vi "AudioTest.Discrete Swept-Sine Measurements (Finite)_V2.vi"() -> ()   [LabVIEW 2018]
doc: "Overview:\nThis VI demonstrates simultaneous frequency response, level, and distortion measurements using a discrete swept-sine technique. This example implements analog input and analog output with 'Finite Samples' sample mode which minimizes sensitivity to bandwidth issues that can cause run-time errors when performing continuous measurements. This VI also demonstrates how finite acquisitions can be read in a single large block or in a series of smaller reads.\n\nRequirements:\nLabVIEW Full Development System\nSound and Vibration Toolkit\n\nInstructions:\n1. Connect the DUT to the DSA device.\n2. Select the AO excitation channel, AI stimulus channel, and AI response channel.\n3. Run the VI.\n\nDetails:\nThis VI performs a swept sine measurement to obtain the root-mean-square (RMS) levels of the acquired stimulus and response, the frequency response of the device under test (DUT), and the harmonic distortion on the response channel. You specify the source and measurement parameters, and the swept sine VIs handle all the DAQ-specific controls required to perform the measurement. You have direct control over the source, input, averaging, and display parameters. You also specify the engineering units to use for the swept sine measurements.\n\nYou can view the time records of the acquired stimulus and response signals. From these graphs, you can see that the transition to the next test frequency always occurs at a zero crossing to minimize non-linear disturbances to the DUT. The RMS levels, frequency response, and harmonic distortion are shown on different tabs."
uses:
  <vilib>/Utility/error.llb/DialogType.ctl
  <vilib>/addons/_NISVFA/_Generation/Signal Generation/SV Signal/SV Signal.lvclass/SV Signal.ctl
  <vilib>/addons/_NISVFA/_Generation/Signal Generation/SV Discrete Sweep/SV Discrete Sweep.lvclass/SV Discrete Sweep.ctl
  <vilib>/addons/Sound and Vibration/svt_Level/SVL AC & DC Level (Time) (1 Ch).vi
  <vilib>/addons/_NISVFA/_Shared subVIs/Common/SV Append Data (N Ch) (DBL).vi
  <vilib>/addons/_NISVFA/_Generation/Signal Generation/SV Signal/Write Leading Synchronization Pulse Enable.vi
  <vilib>/addons/_NISVFA/_Generation/Signal Generation/SV Discrete Sweep/Read All Frequencies and Amplitudes.vi
  <vilib>/addons/_NISVFA/_Generation/Signal Generation/SV Discrete Sweep/Write All Frequencies and Amplitudes.vi
  <vilib>/addons/_NISVFA/_Shared subVIs/Common/svc_Get SV Channel Info.vi
  <vilib>/Analysis/baseanly.llb/Mean.vi
  <vilib>/Analysis/baseanly.llb/Mean (DBL).vi
  <vilib>/addons/_NISVFA/_Shared subVIs/Windowing/svfa_Scaled Time Domain Window (Array).vi
  <vilib>/addons/_NISVFA/_Generation/Signal Generation/SV Discrete Sweep/Read Frequencies and Amplitudes.vi
  <vilib>/Analysis/4window.llb/Force Window.vi
  <vilib>/Analysis/4window.llb/Force Window (DBL).vi
  <vilib>/Analysis/4window.llb/Exponential Window.vi
  <vilib>/Analysis/4window.llb/Exponential Window (DBL).vi
  <vilib>/addons/_NISVFA/_Generation/Signal Generation/SV Discrete Sweep/SV Discrete Sweep.lvclass
  C:/Program Files (x86)/National Instruments/LabVIEW 2018/vi.lib/addons/_NISVFA/_Generation/Signal Generation/SV Signal/SV Signal.lvclass
  C:/Program Files (x86)/National Instruments/LabVIEW 2018/vi.lib/addons/_NISVFA/_Generation/Signal Generation/SV Function/SV Function.lvclass
  <vilib>/addons/_NISVFA/_Generation/Signal Generation/SV Discrete Sweep/Configure Frequency Sweep at Constant Amplitude.vi
  <vilib>/addons/_NISVFA/_Generation/Signal Generation/SV Signal/Write Ramp Parameters.vi
  <vilib>/addons/_NISVFA/_Generation/Signal Generation/SV Signal/Write DC Offset.vi
  <vilib>/addons/_NISVFA/_Generation/Signal Generation/SV Signal/Write Measurement Duration.vi
  <vilib>/addons/_NISVFA/_Generation/Signal Generation/SV Function/Write Measurement Cycles.vi
  <vilib>/addons/_NISVFA/_Generation/Signal Generation/SV Signal/Write Pre-Measurement Settling Duration.vi
  <vilib>/addons/_NISVFA/_Generation/Signal Generation/SV Function/Write Pre-Measurement Settling Cycles.vi
  <vilib>/addons/_NISVFA/_Generation/Signal Generation/SV Signal/Write Sample Rate.vi
  <vilib>/addons/_NISVFA/_Shared subVIs/Data Objects/Waveforms (DBL)/SV Read Next Measurement Data.vi
  <vilib>/addons/_NISVFA/_Shared subVIs/Common/svc_Get Window Info.vi
  <vilib>/addons/_NISVFA/_Shared subVIs/Common/svc_Unit Label to Engineering Units.vi
  <vilib>/addons/_NISVFA/_Shared subVIs/Common/svc_Engineering Units to Unit Label.vi
  <vilib>/addons/_NISVFA/_Spectrum Processing/subVIs/svfa_Spectrum Info Window to windowTd Type Def.vi
  <vilib>/Analysis/0measdsp.llb/Scaled Time Domain Window.vi
  <vilib>/Analysis/0measdsp.llb/Scaled Time Domain Window (DBL).vi
  <vilib>/Utility/error.llb/Error Cluster From Error Code.vi
  <vilib>/Analysis/baseanly.llb/Std Deviation and Variance.vi
  <vilib>/addons/_NISVFA/_Shared subVIs/Common/svc_Caller VI Returned in Error Source.vi
  <vilib>/addons/Sound and Vibration/svt_Single Tone Measurements/SVT Gain and Phase (Time).vi
  <vilib>/addons/Sound and Vibration/svt_Distortion/SVT THD and Harmonic Components (Frequency) (1 Ch).vi
  <vilib>/addons/_NISVFA/_Generation/Signal Generation/SV Signal/SV Signal.lvclass
  <vilib>/addons/_NISVFA/_Shared subVIs/Data Objects/Waveforms (DBL)/Waveforms (N Ch).lvclass
  <vilib>/addons/Sound and Vibration/svt_Distortion/SoundVib_Distortion.lvlib
  <vilib>/addons/Sound and Vibration/svt_Single Tone Measurements/SoundVib_SingleTone.lvlib
  Program Files (x86)/National Instruments/LabVIEW 2018/examples/Sound and Vibration/SoundVib_Audio Examples.lvlib
  C:/Program Files (x86)/National Instruments/LabVIEW 2018/vi.lib/addons/_NISVFA/_Generation/Signal Generation/SV Sinusoid/SV Sinusoid.lvclass
panel:
  in  "volume":dbl=40.0 format="%#_13g"
  in  "Play Cal Output":bool
  in  "Speaker Cal":path=path "C:/MTE/Utah Core Audio Test/Config/Speaker Calibration, PN XXX, SN YYY, v10-30-18.csv"
  out "Cal Speaker Out":waveform(dbl)(graph)
  out "Raw Mic":waveform(dbl)(graph)
  out "Mic dt":dbl
  out "Play dt":dbl
  out "Size Play":i32
  out "Size Mic":i32
  out "Data Cnt":i32
  out "Error":errorcluster
  out "Audio Error":errorcluster
  out "test time":u32
  in  "sweep settings":T1(tab)
  in  "device In":u32
  in  "device Out":u32=1
  in  "Samples/Sec":dbl=51200.0
  in  "Dur(s)":dbl=2.0 format="%.2p"
  out "CalcDur(s)":dbl=1.0 format="%.2p"
  in  "number of steps":i32=190 min=1
  in  "DC offset [V]":dbl format="%.2f"
  in  "amplitude [V]":dbl=1.0 format="%.2p"
  in  "frequency spacing":enum16{"Linear", "Logarithmic"}(ring)=enum."Logarithmic"
  in  "sweep range":cluster{"start":dbl, "stop":dbl}={"start"=20000.0, "stop"=100.0} {"stop" min=0.0 format="%.2f"; "start" min=0.0 format="%.2f"}
  in  "measurement":cluster{"time":dbl, "cycles":dbl}={"time"=0.001, "cycles"=10.0} {"cycles" min=5.0 max=1000.0 step=1.0; "time" min=0.0 max=5.0 step=0.0001 format="%.3f s"}
  in  "settling":cluster{"time":dbl, "cycles":dbl}={"time"=0.0, "cycles"=1.0} {"cycles" min=0.0 max=100.0 step=0.5; "time" min=0.0 max=5.0 step=0.0001 format="%.3f s"}
  in  "views":T2(tab)
  out "Response":waveform(dbl)[](graph)
  out "Stimulus":waveform(dbl)[](graph)
  out "RMS level (response)":cluster{"frequency":dbl[], "magnitude":dbl[]}(graph)
  out "RMS level (stimulus)":cluster{"frequency":dbl[], "magnitude":dbl[]}(graph)
  out "Phase":cluster{"frequency":dbl[], "magnitude":dbl[]}(graph)
  out "Magnitude":cluster{"frequency":dbl[], "magnitude":dbl[]}(graph)
  out "Harmonics":cluster{"f":dbl[], "H_i":dbl[]}[](graph)
  out "THD":cluster{"frequency":dbl[], "THD":dbl[]}(graph)
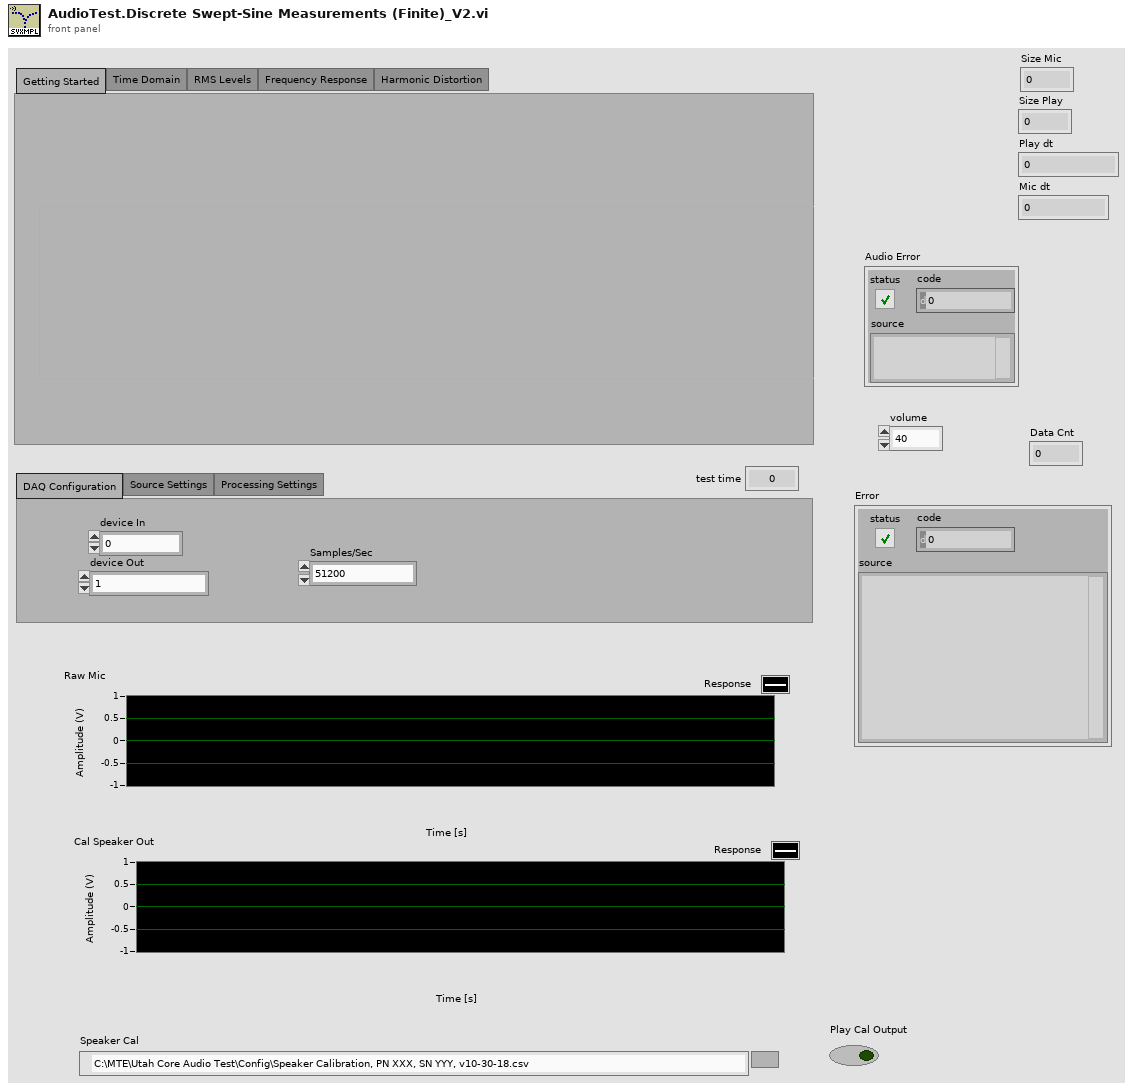
[diagram p1: front panel]
types:
  T1 = enum32{"DAQ Configuration", "Source Settings", "Processing Settings"}
  T2 = enum32{"Getting Started", "Time Domain", "RMS Levels", "Frequency Response", "Harmonic Distortion"}
  T3 = typedef "DialogType.ctl" = u16
  T4 = cluster{"profile":enum16{"Linear", "Half cosine"}, "durations [s]":cluster{"ramp-up":dbl, "transition":dbl, "ramp-down":dbl}}
  T5 = cluster{"frequency [Hz]":dbl, "amplitude [V]":dbl}[]
  T6 = cluster{"gain units":enum16{"dB", "linear ratio"}, "phase units":enum16{"deg", "rad"}, "detected tone stimulus amplitude units":enum16{"EU rms", "EU peak", "EU peak-peak"}, "detected tone response amplitude units":enum16{"EU rms", "EU peak", "EU peak-peak"}}
  T7 = cluster{"THD units":enum16{"dB", "linear ratio", "%"}, "harmonic component amplitude units":enum16{"EU rms", "EU peak", "EU peak-peak", "dB ref fund"}, "detected fundamental amplitude units":enum16{"EU rms", "EU peak", "EU peak-peak"}}
  T8 = typedef "svc_Spectrum Info.ctl" = cluster{"channel name":string, "description":string, "x-axis units":T9, "spectral info":cluster{"spectrum type":T10, "linear/dB":enum16{"linear", "dB"}, "window":u16, "window size":i32, "FFT size":i32}, "engineering units":T11, "custom label":string, "dB reference [EU]":dbl, "peak units":enum16{"rms", "peak", "peak-peak"}, "weighting filter":T12, "spectral density?":bool, "unit label":string, "spectrum skewed?":bool, "complimentary spectrum units":T13}
  T9 = typedef "svc_X-Axis Units.ctl" = u16
  T10 = typedef "svc_Spectrum Type.ctl" = enum16{"FFT Spectrum [complex]", "Amplitude [Magnitude]", "Power [Magnitude^2]", "Cross Spectrum [complex]", "Frequency Response [Complex]"}
  T11 = typedef "svc_Engineering Units Text Ring.ctl" = u16
  T12 = typedef "svc_Weighting Filter Text Ring.ctl" = u16
  T13 = typedef "svc_Complimentary Spectrum Units.ctl" = enum16{"none", "radians", "degrees", "cycles", "imaginary"}
  T14 = cluster{"complex spectrum response":cluster{"f0":dbl, "df":dbl, "complex spectrum":cdb[]}, "spectrum info":T8}
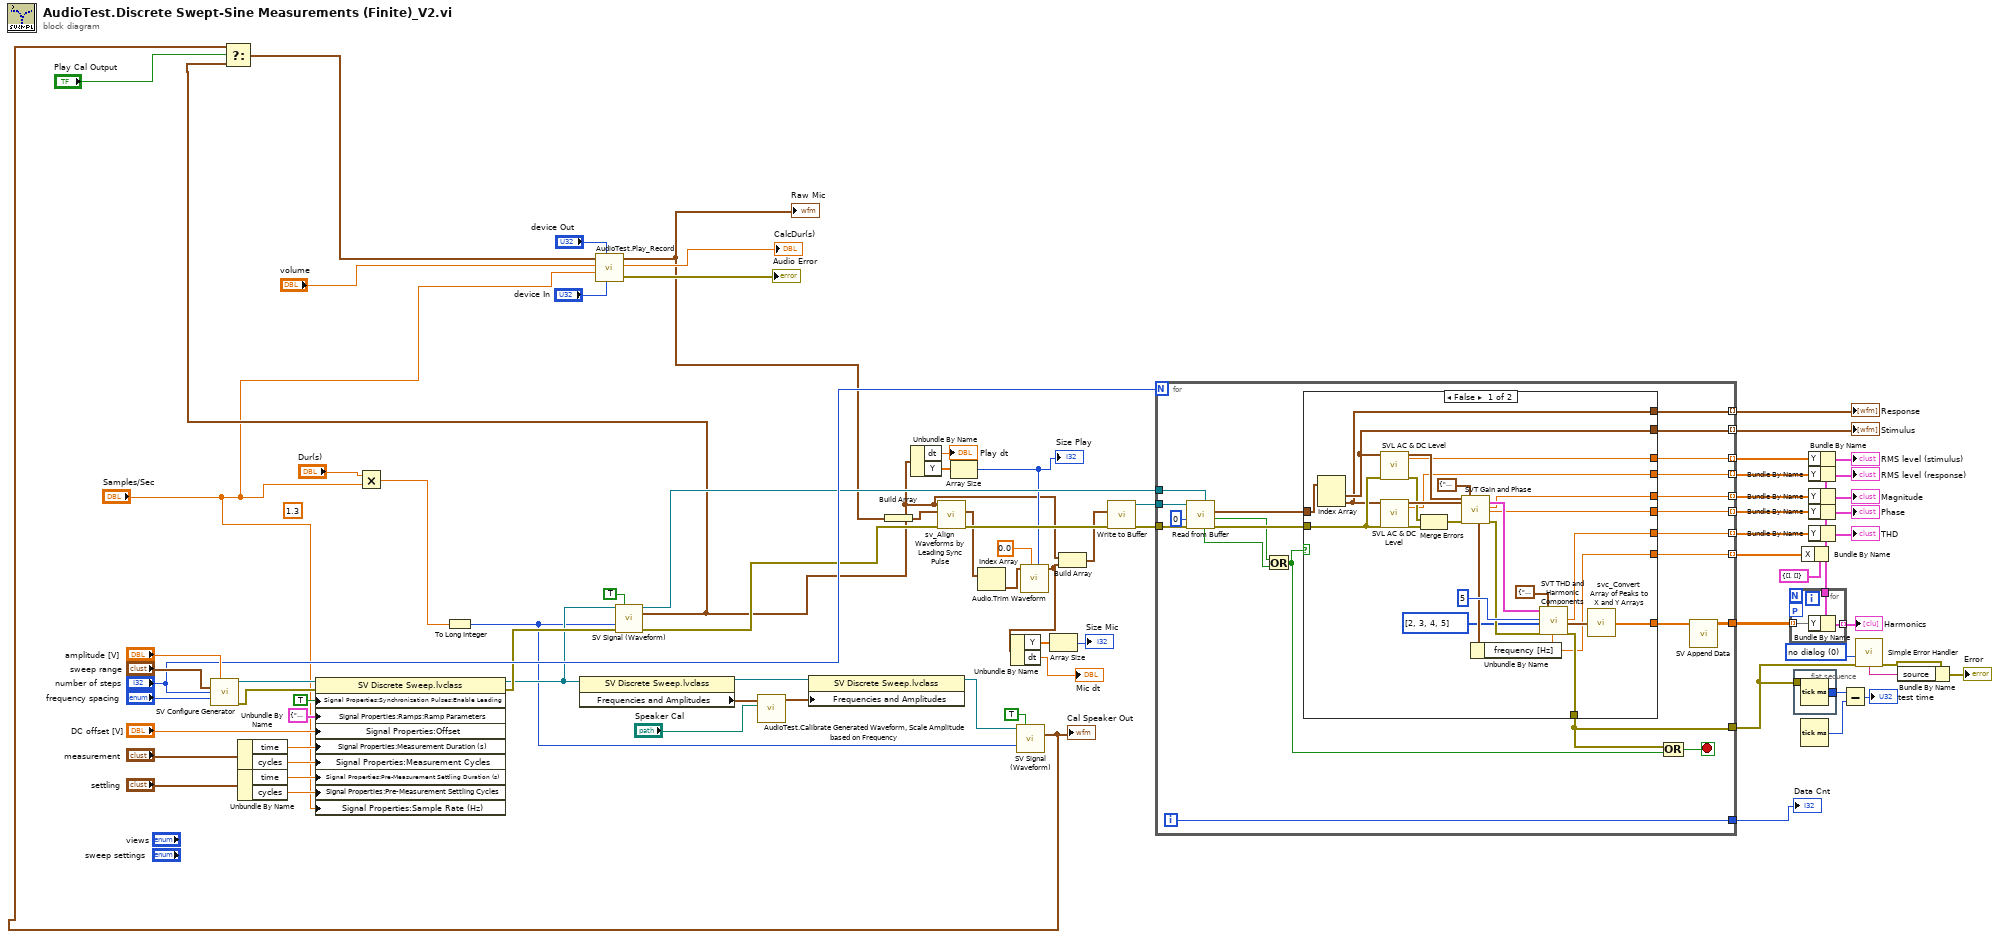
[diagram p0: block diagram]
diagram:
  w31 = T3 0 items=["no dialog", "OK message", "continue or stop message", "OK message + warnings", "continue/stop + warnings"] ("type of dialog (OK msg:1)")
  (unwired) 1.3 ("y")
  n1 = call-poly <vilib>:"SV Configure Generator.vi"("amplitude"="amplitude [V]", "frequency range [Hz]"="sweep range", "number of steps"="number of steps", "profile"="frequency spacing") -> ("signal configuration"=w81:refnum<class "SV Discrete Sweep.lvclass">, "error out"=w70:errorcluster)  [unwired: 10 in]
  n2 = Unbundle By Name("measurement") -> ("time"=w77:dbl, "cycles"=w76:dbl)
  n3 = Unbundle By Name("settling") -> ("time"=w79:dbl, "cycles"=w78:dbl)
  n4 = property class="SV Discrete Sweep.lvclass"(reference=w81, error in=w70, "Signal Properties:Synchronization Pulses:Enable Leading"=TRUE ("Synchronization Pulses:Enable Leading"), "Signal Properties:Ramps:Ramp Parameters"=T4 {"profile"=enum."Half cosine", "durations [s]"={"ramp-up"=0.01, "transition"=0.0, "ramp-down"=0.01}} ("Ramp Parameters"), "Signal Properties:Offset"="DC offset [V]", "Signal Properties:Measurement Duration (s)"=w77, "Signal Properties:Measurement Cycles"=w76, "Signal Properties:Pre-Measurement Settling Duration (s)"=w79, "Signal Properties:Pre-Measurement Settling Cycles"=w78, "Signal Properties:Sample Rate (Hz)"="Samples/Sec") -> (reference out=w19:refnum<class "SV Discrete Sweep.lvclass">, error out=w41:errorcluster)
  n5 = Multiply(x="Dur(s)", y="Samples/Sec") -> (x*y=w20:dbl)
  n6 = To Long Integer(number=w20) -> (32bit integer=w13:i32)
  n7 = property class="SV Discrete Sweep.lvclass"(reference=w19) -> (reference out=w16:refnum<class "SV Discrete Sweep.lvclass">, "Frequencies and Amplitudes"=w18:T5)  [unwired: 1 in, 1 out]
  n8 = call-dynamic "SV Signal (Waveform).vi"("signal configuration"=w19, "reset"=TRUE, "samples"=w13, "error in (no error)"=w41) -> ("signal configuration"=w40:refnum<class "SV Discrete Sweep.lvclass">, "output waveform"=w9:waveform(dbl), "error out"=w39:errorcluster)  [unwired: 6 in, 3 out]
  n9 = call "AudioTest.Calibrate Generated Waveform, Scale Amplitude based on Frequency.vi"("Calibration File"="Speaker Cal", "Frequencies and Amplitudes"=w18) -> ("Frequencies and Amplitudes Out"=w17:T5)  [unwired: 8 in, 1 out]
  n10 = property class="SV Discrete Sweep.lvclass"(reference=w16, "Frequencies and Amplitudes"=w17) -> (reference out=w14:refnum<class "SV Discrete Sweep.lvclass">)  [unwired: 1 in, 1 out]
  n11 = Unbundle By Name(w9) -> ("dt"=→"Play dt":dbl, "Y"=w32:dbl[])
  n12 = Array Size(array=w32) -> (size(s)=w24:i32)
  "Size Play" <- w24
  n13 = call-dynamic "SV Signal (Waveform).vi"("signal configuration"=w14, "reset"=TRUE, "samples"=w13) -> ("output waveform"=w11:waveform(dbl))  [unwired: 7 in, 5 out]
  "Cal Speaker Out" <- w11
  n14 = Select(t=w11, s="Play Cal Output", f=w9) -> (s? t:f=w6:waveform(dbl))
  n15 = call "AudioTest.Play_Record.vi"("Record Device ID"="device In", "Play Device ID"="device Out", "Sample Rate (Hz)"="Samples/Sec", "volume"="volume", "Stimulus Wvfrm"=w6) -> ("Error Out"=→"Audio Error":errorcluster, "PlayDur(s)"=→"CalcDur(s)":dbl, "Recorded Wvfrm"=w1:waveform(dbl))  [unwired: 4 in]
  "Raw Mic" <- w1
  n16 = Build Array(w1) -> (w37:waveform(dbl)[])
  n17 = call "sv_Align Waveforms by Leading Sync Pulse.vi"("error in (no error)"=w39, "response signals"=w37, "alignment reference signal"=w9) -> ("error out"=w43:errorcluster, "aligned signals"=w35:waveform(dbl)[])  [unwired: 4 in, 3 out]
  n18 = Index Array(array=w35) -> (element=w36:waveform(dbl))  [unwired: 1 in]
  n19 = call "Audio.Trim Waveform.vi"("Len"=w24, "Max Delay"=0.0, "Data In"=w36) -> ("Data Out"=w26:waveform(dbl))  [unwired: 8 in]
  n20 = Unbundle By Name(w26) -> ("Y"=w27:dbl[], "dt"=→"Mic dt":dbl)
  n21 = Array Size(array=w27) -> (size(s)=→"Size Mic":i32)
  n22 = Build Array(w9, w26) -> (w34:waveform(dbl)[])
  n23 = call <vilib>:"Write to Buffer.vi"("error in (no error)"=w43, "waveforms"=w34) -> ("error out"=w44:errorcluster, "buffer out"=w45:refnum<data-value>)  [unwired: 7 in, 1 out]
  n24 = for {
    N: "number of steps" -> [_]
    tunnel: w45 -> [w101]
    tunnel: w40 -> [w100]
    tunnel: w44 -> [w99]
    tunnel: [w87] -> w50
    tunnel: [w96] -> w62 mode=indexing
    tunnel: [w95] -> w61 mode=indexing
    tunnel: [w94] -> w60 mode=indexing
    tunnel: [w93] -> w59 mode=indexing
    tunnel: [w92] -> w58 mode=indexing
    tunnel: [w83] -> w54 mode=indexing
    tunnel: [w90] -> w53
    tunnel: [w89] -> w52 mode=indexing
    tunnel: [w88] -> w51 mode=indexing
    tunnel: [w84] -> w21
    i -> [w84]
    stop <- w97 stop-if-true
    n25 = call-poly <vilib>:"Read from Buffer.vi"("test signal configuration"=w100, "error in (no error)"=w99, "timeout (1000 ms)"=0, "buffer"=w101) -> ("error out"=w103:errorcluster, "end of buffer"=w86:bool, "waveforms subset"=w98:waveform(dbl)[], "done"=w85:bool)  [unwired: 3 in, 1 out]
    n26 = Or(x=w86, y=w85) -> (x .or. y?=w82:bool)
    n27 = case shown="False" w82 {
      tunnel: w103 -> [w128 _]
      tunnel: w98 -> [w127 _]
      tunnel: [w113 _] -> w96
      tunnel: [w112 _] -> w95
      tunnel: [w111 _] -> w94
      tunnel: [w110 _] -> w93
      tunnel: [w109 _] -> w92
      tunnel: [w108 _] -> w91
      tunnel: [w107 _] -> w89
      tunnel: [w106 _] -> w88
      tunnel: [w105 _] -> w87
      tunnel: [w104 _] -> w83
      frame False {
        n28 = Index Array(array=w127) -> (element #1=w107:waveform(dbl), element #2=w106:waveform(dbl))  [unwired: 2 in]
        n29 = call-poly <vilib>:"SVL AC & DC Level.vi"("scaled signal [EU]"=w107, "error in (no error)"=w128) -> ("AC signal [EU]"=w121:waveform(dbl), "AC level [EU rms]"=w113:dbl, "error out"=w118:errorcluster)  [unwired: 12 in, 3 out]
        n30 = call-poly <vilib>:"SVL AC & DC Level.vi"("scaled signal [EU]"=w106, "error in (no error)"=w128) -> ("AC signal [EU]"=w120:waveform(dbl), "AC level [EU rms]"=w112:dbl, "error out"=w117:errorcluster)  [unwired: 12 in, 3 out]
        n31 = Merge Errors(w118, w117) -> (w116:errorcluster)
        n32 = call-poly <vilib>:"SVT Gain and Phase.vi"("stimulus signal X [EUx]"=w121, "response signal Y [EUy]"=w120, "error in (no error)"=w116, "desired units"=T6 {"gain units"=enum."dB", "phase units"=enum."deg", "detected tone stimulus amplitude units"=enum."EU rms", "detected tone response amplitude units"=enum."EU rms"}) -> ("detected tone response"=w115:cluster{"frequency [Hz]":dbl, "amplitude":dbl}, "complex spectrum\nresponse Y"=w122:T14, "gain"=w111:dbl, "phase lag"=w110:dbl, "error out"=w119:errorcluster)  [unwired: 8 in, 3 out]
        n33 = Unbundle By Name(w115) -> ("frequency [Hz]"=w104:dbl)
        n34 = call-poly <vilib>:"SVT THD and Harmonic Components.vi"("complex spectrum"=w122, "maximum harmonic"=5, "harmonics to visualize"=i32[] [2, 3, 4, 5], "error in (no error)"=w119, "desired units"=T7 {"THD units"=enum."dB", "harmonic component amplitude units"=enum."dB ref fund", "detected fundamental amplitude units"=enum."EU peak"}, "expected fundamental frequency [Hz]"=w104) -> ("THD"=w109:dbl, "harmonic components"=w123:cluster{"frequency [Hz]":dbl, "amplitude":dbl}[], "error out"=w105:errorcluster)  [unwired: 6 in, 5 out]
        n35 = call <vilib>:"svc_Convert Array of Peaks to X and Y Arrays.vi"("peaks"=w123) -> ("Y"=w108:dbl[])  [unwired: 3 in, 1 out]
      }
      frame True {
      }
    }
    n36 = Compound Arithmetic op=OR(w87, w82) -> (w97:bool)
    n37 = call-poly <vilib>:"SV Append Data.vi"("data in"=w91) -> ("appended data"=w90:dbl[][])  [unwired: 10 in]
  }
  "Stimulus" <- w52
  "Response" <- w51
  "Data Cnt" <- w21
  n38 = flat-sequence {
    tunnel: w50 -> [_]
    tunnel: [w129] -> w49
    frame #0 {
      n39 = Tick Count (ms)() -> (millisecond timer value=w129:u32)
    }
  }
  n40 = Tick Count (ms)() -> (millisecond timer value=w47:u32)
  n41 = Bundle By Name(cluster=cluster{"X":dbl[], "Y":dbl[]} {"X"=[], "Y"=[]} ("THD vs Amplitude"), "X"=w54) -> (w55:cluster{"X":dbl[], "Y":dbl[]})
  n42 = for {
    tunnel: [w132] -> w57 mode=indexing
    tunnel: w55 -> [w131]
    workers-P: _ -> [_]
    tunnel: w53 -> [w130] mode=indexing
    n43 = Bundle By Name(cluster=w131, "Y"=w130) -> (w132:cluster{"X":dbl[], "Y":dbl[]})
  }
  "Harmonics" <- w57
  n44 = Bundle By Name(cluster=w55, "Y"=w62) -> (→"RMS level (stimulus)":cluster{"X":dbl[], "Y":dbl[]})
  n45 = Bundle By Name(cluster=w55, "Y"=w61) -> (→"RMS level (response)":cluster{"X":dbl[], "Y":dbl[]})
  n46 = Bundle By Name(cluster=w55, "Y"=w60) -> (→"Magnitude":cluster{"X":dbl[], "Y":dbl[]})
  n47 = Bundle By Name(cluster=w55, "Y"=w59) -> (→"Phase":cluster{"X":dbl[], "Y":dbl[]})
  n48 = Bundle By Name(cluster=w55, "Y"=w58) -> (→"THD":cluster{"X":dbl[], "Y":dbl[]})
  n49 = Subtract(x=w49, y=w47) -> (x-y=→"test time":u32)
  n50 = call <vilib>:"Simple Error Handler.vi"("type of dialog (OK msg:1)"=w31, "error in (no error)"=w50) -> ("error out"=w30:errorcluster, "message"=w29:string)  [unwired: 3 in, 3 out]
  n51 = Bundle By Name(cluster=w30, "source"=w29) -> (→"Error":errorcluster)
